vi "GV.vi"(1 "OK Button":bool, 2 "Vmin":dbl, 3 "Vmax":dbl, 4 "dV":dbl, 5 "Vo":dbl) -> (0 "Waveform Graph":dbl[](graph))   [LabVIEW 2011]
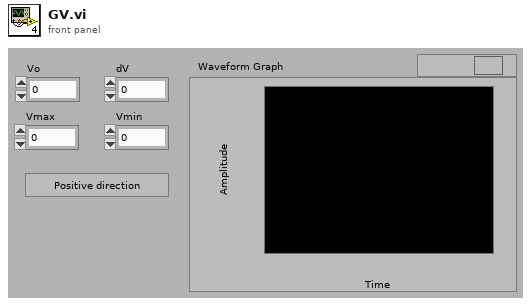
[diagram p1: front panel]
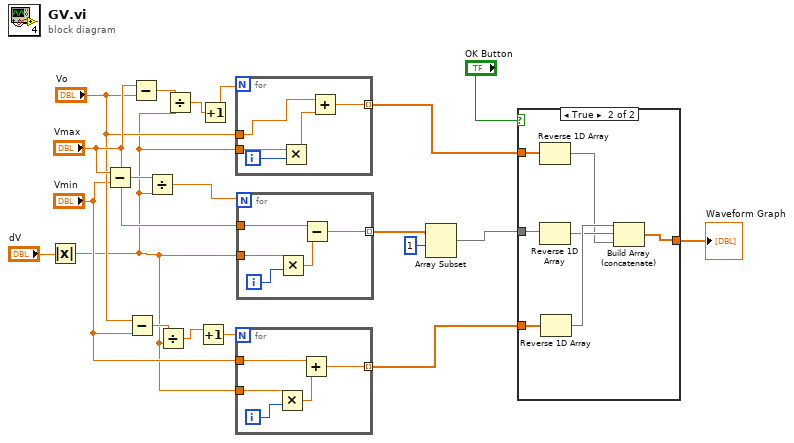
[diagram p0: block diagram]
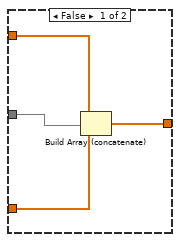
[diagram p2: hidden frame]
diagram:
  n1 = Absolute Value(x="dV") -> (abs(x)=w1:dbl)
  n2 = Subtract(x="Vmax", y="Vmin") -> (x-y=w16:dbl)
  n3 = Subtract(x="Vo", y="Vmin") -> (x-y=w13:dbl)
  n4 = Subtract(x="Vmax", y="Vo") -> (x-y=w19:dbl)
  n5 = Divide(x=w16, y=w1) -> (x/y=w6:dbl)
  n6 = Divide(x=w13, y=w1) -> (x/y=w12:dbl)
  n7 = Divide(x=w19, y=w1) -> (x/y=w18:dbl)
  n8 = Increment(x=w12) -> (x+1=w11:dbl)
  n9 = Increment(x=w18) -> (x+1=w17:dbl)
  n10 = for {
    N: w17 -> [_]
    tunnel: "Vo" -> [w25]
    tunnel: w1 -> [w23]
    tunnel: [w21] -> w9 mode=indexing
    i -> [w24]
    n11 = Multiply(x=w23, y=w24) -> (x*y=w22:dbl)
    n12 = Add(x=w25, y=w22) -> (x+y=w21:dbl)
  }
  n13 = for {
    N: w11 -> [_]
    tunnel: "Vmin" -> [w30]
    tunnel: w1 -> [w28]
    tunnel: [w26] -> w8 mode=indexing
    i -> [w29]
    n14 = Multiply(x=w28, y=w29) -> (x*y=w27:dbl)
    n15 = Add(x=w30, y=w27) -> (x+y=w26:dbl)
  }
  n16 = for {
    N: w6 -> [_]
    tunnel: "Vmax" -> [w35]
    tunnel: w1 -> [w33]
    tunnel: [w31] -> w5 mode=indexing
    i -> [w34]
    n17 = Multiply(x=w33, y=w34) -> (x*y=w32:dbl)
    n18 = Subtract(x=w35, y=w32) -> (x-y=w31:dbl)
  }
  n19 = Array Subset(array=w5, index=1) -> (w3:dbl[])  [unwired: 1 in]
  n20 = case shown="True" "OK Button" {
    tunnel: w9 -> [w39 w44]
    tunnel: w3 -> [w38 w45]
    tunnel: w8 -> [w37 w46]
    tunnel: [w36 w40] -> w7
    frame False {
      n21 = Build Array (concatenate)(w39, w38, w37) -> (w36:dbl[])
    }
    frame True {
      n22 = Reverse 1D Array(array=w44) -> (reversed array=w41:dbl[])
      n23 = Reverse 1D Array(array=w45) -> (reversed array=w42:dbl[])
      n24 = Reverse 1D Array(array=w46) -> (reversed array=w43:dbl[])
      n25 = Build Array (concatenate)(w43, w42, w41) -> (w40:dbl[])
    }
  }
  "Waveform Graph" <- w7
